vi "Configure Transient Operation.vi"(0 "VISA resource name":refnum<visa-resource-name>, 1 "B Level Value (2.000)":dbl=2.0 min=0.0 max=7500.0 step=1.0 format="%.3f", 2 "A Width (1s)":dbl=1.0 min=0.0 max=120.0 step=1.0 format="%#.3f", 5 "Transient Mode (0:Continuous)":u16(ring) items=["Continuous", "Pulse", "Toggle"], 7 "Rise Slew Rate  (1)":dbl=1.0 min=0.0 max=7500.0 step=1.0 format="%.3f", 9 "A Level Value (1.000)":dbl=1.0 min=0.0 max=7500.0 step=1.0 format="%.3f", 11 "error in (no error)":errorcluster, 12 "Fall Slew Rate (1)":dbl=1.0 min=0.0 max=7500.0 step=1.0 format="%.3f", 13 "B Width (1s)":dbl=1.0 min=0.0 max=120.0 step=1.0 format="%#.3f") -> (4 "VISA resource name out":refnum<visa-resource-name>, 15 "error out":errorcluster)   [LabVIEW 2024, in "BK Precision 8500B Series.lvlib"]
doc: "Configures the transient load operation between A level and B level and Slew Rate during Transient operation. Selects the type of transient: Continuous, Pulse or Toggled.\n\nNote: The operation mode must be configured first using <b>Configure Operation Mode.vi</b> before running this VI. Transient mode is only available for CC mode."
uses:
  BK Precision 8500B Series.lvlib
panel:
  # "A/us"
  # "A/us"
  # "s"
  # "s"
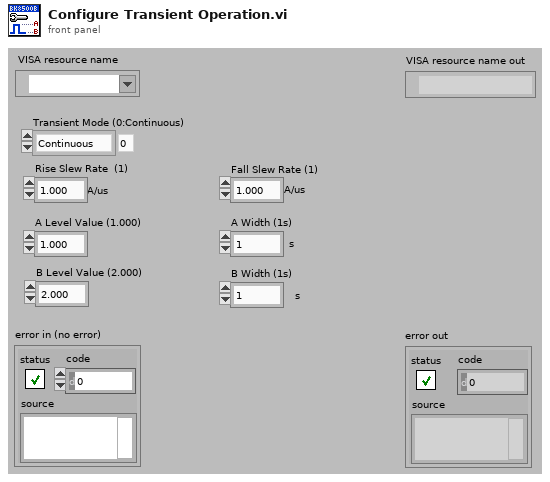
[diagram p1: front panel]
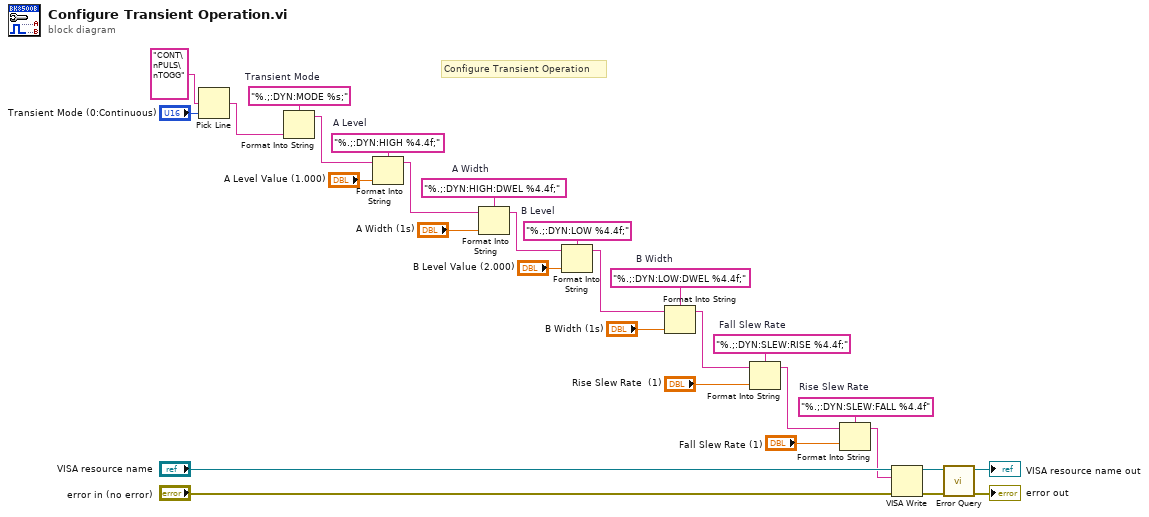
[diagram p0: block diagram]
diagram:
  w5 = "%.;:DYN:SLEW:RISE %4.4f;"  # Fall Slew Rate
  w7 = "%.;:DYN:SLEW:FALL %4.4f"  # Rise Slew Rate
  w9 = "%.;:DYN:LOW:DWEL %4.4f;"  # B Width
  w8 = "%.;:DYN:LOW %4.4f;"  # B Level
  w23 = "%.;:DYN:HIGH:DWEL %4.4f;"  # A Width
  w24 = "%.;:DYN:HIGH %4.4f;"  # A Level
  w25 = "%.;:DYN:MODE %s;"  # Transient Mode
  # "Configure Transient Operation"
  n1 = Pick Line(multi-line string="CONT\nPULS\nTOGG", line index="Transient Mode (0:Continuous)") -> (output string=w16:string)  [unwired: 1 in]
  n2 = Format Into String(format string=w25, w16) -> (resulting string=w21:string)  [unwired: 2 in, 1 out]
  n3 = Format Into String(format string=w24, initial string=w21, "A Level Value (1.000)") -> (resulting string=w20:string)  [unwired: 1 in, 1 out]
  n4 = Format Into String(format string=w23, initial string=w20, "A Width (1s)") -> (resulting string=w12:string)  [unwired: 1 in, 1 out]
  n5 = Format Into String(format string=w8, initial string=w12, "B Level Value (2.000)") -> (resulting string=w11:string)  [unwired: 1 in, 1 out]
  n6 = Format Into String(format string=w9, initial string=w11, "B Width (1s)") -> (resulting string=w6:string)  [unwired: 1 in, 1 out]
  n7 = Format Into String(format string=w5, initial string=w6, "Rise Slew Rate  (1)") -> (resulting string=w2:string)  [unwired: 1 in, 1 out]
  n8 = Format Into String(format string=w7, initial string=w2, "Fall Slew Rate (1)") -> (resulting string=w1:string)  [unwired: 1 in, 1 out]
  n9 = VISA Write(VISA resource name="VISA resource name", write buffer=w1, error in (no error)="error in (no error)") -> (VISA resource name out=w26:refnum<visa-resource-name>, error out=w27:errorcluster)  [unwired: 1 out]
  n10 = call "Error Query.vi"("error in (no error)"=w27, "VISA resource name"=w26) -> ("error out"=→"error out":errorcluster, "VISA resource name out"=→"VISA resource name out":refnum<visa-resource-name>)  [unwired: 6 in, 2 out]
